vi "Stop.vi"(7 "Emergency Stop? (F)":bool, 8 "error in (no error)":errorcluster, 11 "API-Reference in":refnum<k1>) -> (0 "error out":errorcluster, 3 "API-Reference out":refnum<k1>)   [LabVIEW 2018, in "Copy of Actor.lvclass"]
uses:
  Copy of Actor.lvclass
  API-Data.ctl
  Stopped.ctl
  Event-References.ctl
  Stop.ctl
  Launched.ctl
  Some Request.ctl
  Some Response.ctl
  <vilib>/event_ctls.llb/usereventprio.ctl
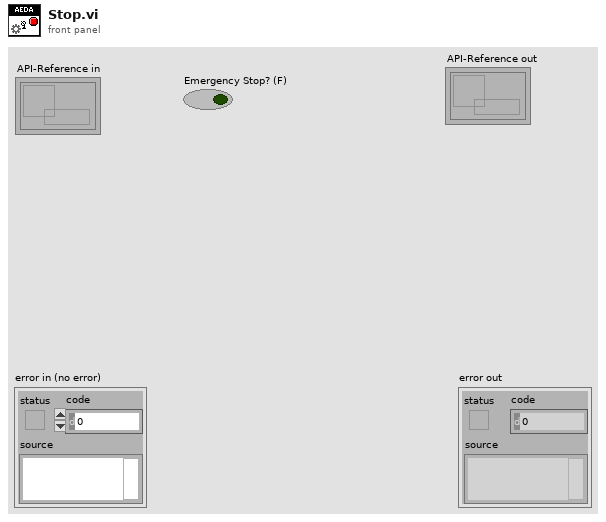
[diagram p1: front panel]
types:
  T1 = typedef "Copy of Actor.lvclass/Stop.ctl" = enum16{"Normal", "Emergency"}
  T2 = typedef "usereventprio.ctl" = enum32{"high priority", "normal priority"}
  T3 = typedef "Copy of Actor.lvclass/API-Data.ctl" = cluster{"Launch":refnum<notifier>, "Stopped":refnum<user-event>, "Actor-Events":T4, "Stopped Registration":refnum<event-registration>}
  T4 = typedef "Copy of Actor.lvclass/Event-References.ctl" = cluster{"Stop":refnum<user-event>, "Launched":refnum<user-event>, "Some Request":refnum<user-event>}
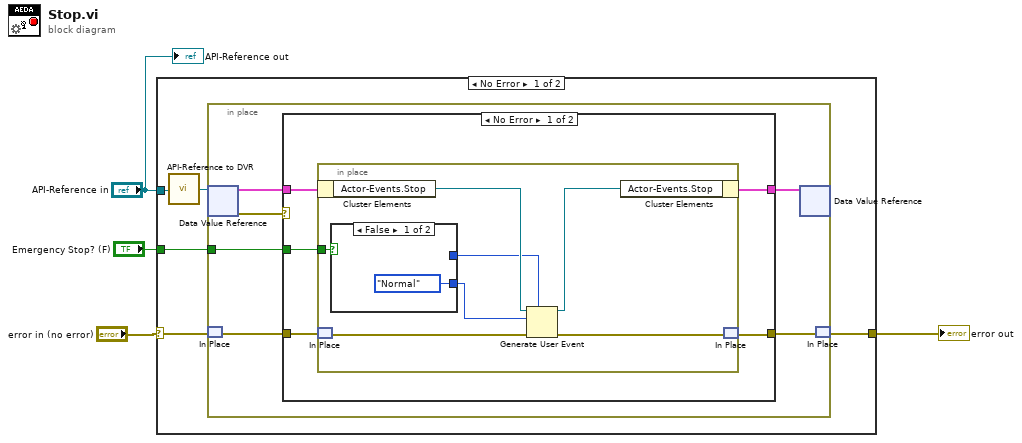
[diagram p0: block diagram]
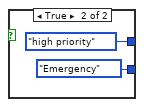
[diagram p2: hidden frame]
diagram:
  n1 = case shown="No Error" "error in (no error)" {
    selector: "error in (no error)" -> [w9 w33]
    tunnel: [w8 w33] -> w2
    tunnel: "API-Reference in" -> [w5 _]
    tunnel: "Emergency Stop? (F)" -> [w7 _]
    frame No Error {
      n2 = call "API-Reference to DVR.vi"("API-Reference in"=w5) -> ("Data Value Reference out"=w6:refnum<data-value>)
      n3 = in-place {
        in-place-border: w7 -> [w10]
        n4 = in-place-dvr #1(w6) -> (w14:T3, w15:errorcluster)
        n5 = in-place-match #2(w9) -> (w12:errorcluster)
        n6 = case shown="No Error" w15 {
          selector: w15 -> [_ w32]
          tunnel: w14 -> [w18 w31]
          tunnel: [w16 w31] -> w13
          tunnel: w12 -> [w20 _]
          tunnel: [w19 w32] -> w11
          tunnel: w10 -> [w17 _]
          frame No Error {
            n7 = in-place {
              in-place-border: w17 -> [w25]
              n8 = in-place-cluster #3(w18) -> ("Actor-Events.Stop"=w26:refnum<user-event>)
              n9 = in-place-match #4(w20) -> (w27:errorcluster)
              n10 = case shown="False" w25 {
                tunnel: [Stop."Normal" ("Stop") Stop."Emergency" ("Stop")] -> w23
                tunnel: [_ usereventprio."high priority" ("priority (normal)")] -> w22
                frame False {
                }
                frame True {
                }
              }
              n11 = Generate User Event(priority (normal)=w22, user event=w26, event data cluster=w23, error in=w27) -> (user event out=w24:refnum<user-event>, error out=w21:errorcluster)
              n12 = in-place-cluster #3("Actor-Events.Stop"=w24) -> (w16:T3)
              n13 = in-place-match #4(w21) -> (w19:errorcluster)
            }
          }
          frame Error {
          }
        }
        n14 = in-place-dvr #1(w13) -> ()  [unwired: 2 out]
        n15 = in-place-match #2(w11) -> (w8:errorcluster)
      }
    }
    frame Error {
    }
  }
  "error out" <- w2
  "API-Reference out" <- "API-Reference in"
